vi "Input data row.vi"(8 "error in (no error)":errorcluster, 10 "Last row of data file":string[](array[string]), 11 "Automatic Mode in":refnum<class "Automatic Mode.lvclass">) -> (0 "error out":errorcluster, 3 "Automatic Mode out":refnum<class "Automatic Mode.lvclass">)   [LabVIEW 2019, in "Automatic Mode.lvclass"]
uses:
  Automatic Mode.lvclass
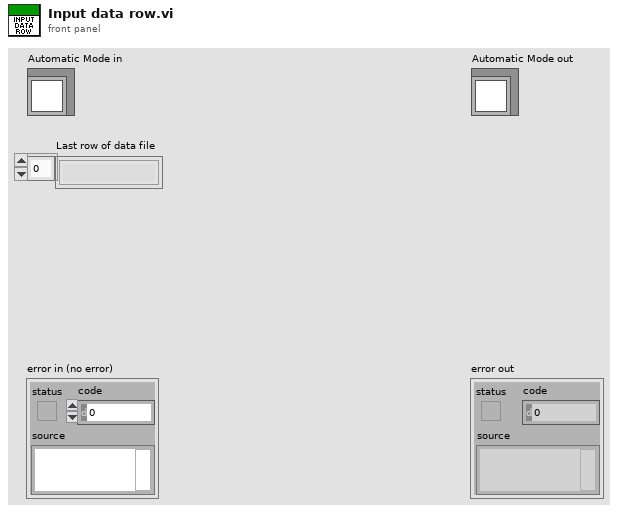
[diagram p1: front panel]
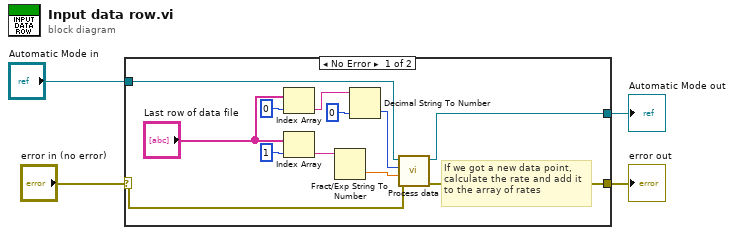
[diagram p0: block diagram]
diagram:
  n1 = case shown="No Error" "error in (no error)" {
    selector: "error in (no error)" -> [w7 w18]
    tunnel: [w5 w18] -> w3
    tunnel: [w6 w17] -> w1
    tunnel: "Automatic Mode in" -> [w10 w17]
    frame No Error {
      # "If we got a new data point,\ncalculate the rate and add it\nto the array of rates"
      n2 = Index Array(array="Last row of data file", index=0) -> (element=w14:string)
      n3 = Index Array(array="Last row of data file", index=1) -> (element=w13:string)
      n4 = Fract/Exp String To Number(string=w13) -> (number=w8:dbl)  [unwired: 3 in, 1 out]
      n5 = Decimal String To Number(string=w14, default (0L)=i64 0 ("default (0 I32)")) -> (number=w9:i64)  [unwired: 1 in, 1 out]
      n6 = call "Process data.vi"("error in (no error)"=w7, "New polarization"=w8, "New eventnum"=w9, "Automatic Mode in"=w10) -> ("error out"=w5:errorcluster, "Automatic Mode out"=w6:refnum<class "Automatic Mode.lvclass">)  [unwired: 5 in, 1 out]
    }
    frame Error {
    }
  }
  "error out" <- w3
  "Automatic Mode out" <- w1
